vi "Close.vi"(8 "error in (no error)":errorcluster, 11 "VISA resource name":refnum<visa-resource-name>) -> (0 "error out":errorcluster)   [LabVIEW 2020, in "CAEN PSM.lvlib"]
doc: "This function terminates the software connection to the instrument."
uses:
  CAEN PSM.lvlib
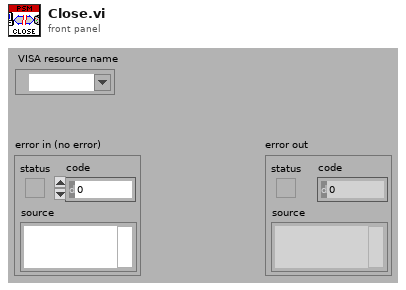
[diagram p1: front panel]
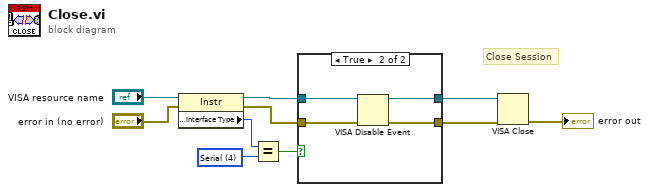
[diagram p0: block diagram]
diagram:
  w8 = u16 4 items=["GPIB"=1, "VXI"=2, "GPIB-VXI"=3, "Serial"=4, "PXI"=5, "TCPIP"=6, "USB"=7] ("Interface Information:Interface Type")
  # "Close Session"
  n1 = property class="Instr"(reference="VISA resource name", error in="error in (no error)") -> (reference out=w1:refnum<visa-resource-name>, error out=w3:errorcluster, "Interface Information:Interface Type"=w9:u16)
  n2 = Equal?(x=w9, y=w8) -> (x = y?=w5:bool)
  n3 = case shown="True" w5 {
    tunnel: [w11 w16] -> w4
    tunnel: w3 -> [w11 w15]
    tunnel: w1 -> [w12 w14]
    tunnel: [w12 w13] -> w2
    frame False {
    }
    frame True {
      n4 = VISA Disable Event(8:w15, 11:w14) -> (0:w16:errorcluster, 3:w13:refnum<visa-resource-name>)  [unwired: 1 in, 1 out]
    }
  }
  n5 = VISA Close(VISA resource name=w2, error in (no error)=w4) -> (error out=→"error out":errorcluster)
